vi "test_libssh2_userauth_keyboard_interactive_ex.vi"() -> ()   [LabVIEW 2013, in "libssh2_integration_tests.lvlib"]
uses:
  libssh2_integration_tests.lvlib
  callback_lvssh2_userauth_keyboard_interactive_response_function.vi
  libssh2/libssh2_init_default.vi
  libssh2/libssh2_session_handshake_tcp.vi
  libssh2/libssh2.lvlib
  <vilib>/addons/_JKI Toolkits/Caraya/classes/Test/Test.lvclass
  <vilib>/addons/_JKI Toolkits/Caraya/classes/Assert/Assert.lvclass
panel:
  out "error out":errorcluster
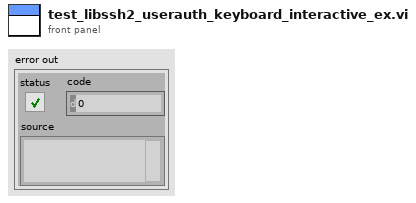
[diagram p1: front panel]
types:
  T1 = typedef "libssh2.lvlib/Session Refnum.ctl" = refnum<k1>
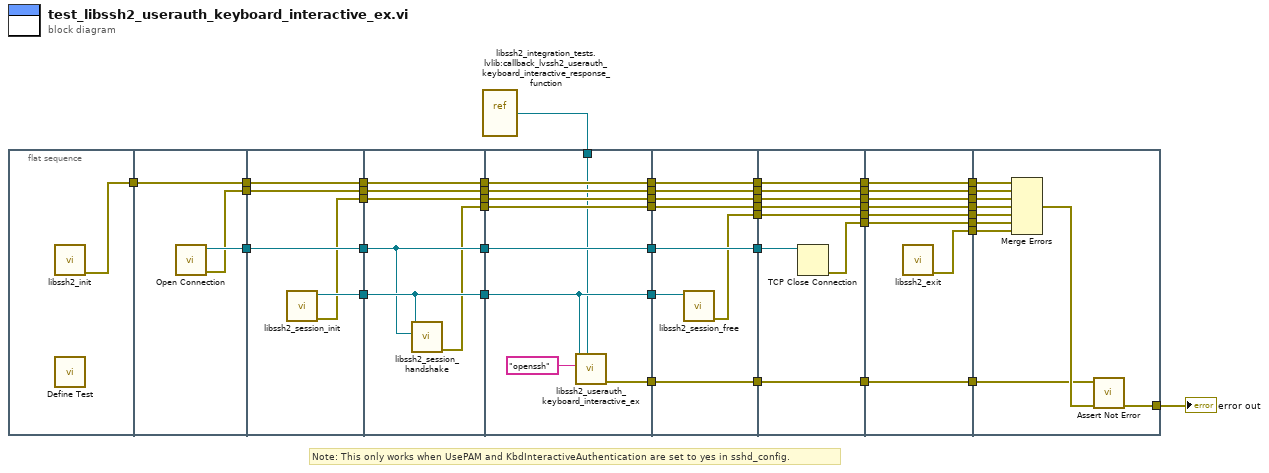
[diagram p0: block diagram]
diagram:
  # "Note: This only works when UsePAM and KbdInteractiveAuthentication are set to yes in sshd_config."
  n1 = flat-sequence {
    tunnel: [w47] -> w46
    tunnel: [w50] -> w45
    tunnel: w46 -> [w49]
    tunnel: [w49] -> w44
    tunnel: [w48] -> w43
    tunnel: w45 -> [w55]
    tunnel: [w55] -> w16
    tunnel: w44 -> [w54]
    tunnel: [w54] -> w15
    tunnel: w43 -> [w53]
    tunnel: [w53] -> w14
    tunnel: [w52] -> w13
    tunnel: [w51] -> w12
    tunnel: w16 -> [w57]
    tunnel: [w57] -> w31
    tunnel: w15 -> [w61]
    tunnel: [w61] -> w30
    tunnel: w14 -> [w60]
    tunnel: [w60] -> w29
    tunnel: [w59] -> w28
    tunnel: w13 -> [w59]
    tunnel: w12 -> [w58]
    tunnel: [w58] -> w27
    tunnel: [w56] -> w26
    tunnel: w31 -> [w70]
    tunnel: [w70] -> w8
    tunnel: w30 -> [w69]
    tunnel: [w69] -> w7
    tunnel: w29 -> [w68]
    tunnel: [w68] -> w6
    tunnel: w28 -> [w65]
    tunnel: w27 -> [w67]
    tunnel: [w67] -> w5
    tunnel: w26 -> [w66]
    tunnel: [w66] -> w4
    tunnel: [w65] -> w3
    tunnel: [w63] -> w2
    tunnel: w1 -> [w62]
    tunnel: w8 -> [w78]
    tunnel: [w78] -> w25
    tunnel: w7 -> [w77]
    tunnel: [w77] -> w24
    tunnel: w6 -> [w76]
    tunnel: [w76] -> w23
    tunnel: w5 -> [w75]
    tunnel: [w75] -> w22
    tunnel: w4 -> [w74]
    tunnel: [w74] -> w21
    tunnel: [w73] -> w18
    tunnel: [w72] -> w9
    tunnel: w2 -> [w72]
    tunnel: w3 -> [w71]
    tunnel: w25 -> [w86]
    tunnel: w24 -> [w85]
    tunnel: [w85] -> w42
    tunnel: w23 -> [w84]
    tunnel: [w84] -> w41
    tunnel: [w83] -> w40
    tunnel: w22 -> [w82]
    tunnel: [w82] -> w39
    tunnel: w21 -> [w81]
    tunnel: [w81] -> w38
    tunnel: [w80] -> w19
    tunnel: w18 -> [w80]
    tunnel: [w79] -> w10
    tunnel: w9 -> [w79]
    tunnel: w42 -> [w94]
    tunnel: [w94] -> w37
    tunnel: w41 -> [w93]
    tunnel: [w93] -> w36
    tunnel: w40 -> [w92]
    tunnel: [w92] -> w35
    tunnel: [w91] -> w34
    tunnel: w39 -> [w90]
    tunnel: [w90] -> w33
    tunnel: w38 -> [w89]
    tunnel: [w89] -> w32
    tunnel: [w88] -> w20
    tunnel: w19 -> [w88]
    tunnel: [w87] -> w11
    tunnel: w10 -> [w87]
    tunnel: w37 -> [w104]
    tunnel: w36 -> [w103]
    tunnel: w35 -> [w102]
    tunnel: w34 -> [w101]
    tunnel: w33 -> [w100]
    tunnel: [w98] -> w17
    tunnel: w32 -> [w97]
    tunnel: w20 -> [w96]
    tunnel: w11 -> [w95]
    frame #0 {
      n2 = call-poly "libssh2_init.vi"() -> ("error out"=w47:errorcluster)  [unwired: 11 in]
      n3 = call <vilib>:"Define Test.vi"() -> ()  [unwired: 10 in, 2 out]
    }
    frame #1 {
      n4 = call "Open Connection.vi"() -> ("error out"=w48:errorcluster, "connection ID"=w50:refnum<k5>)  [unwired: 10 in]
    }
    frame #2 {
      n5 = call "libssh2_session_init.vi"() -> ("error out"=w51:errorcluster, "session"=w52:T1)  [unwired: 10 in]
    }
    frame #3 {
      n6 = call-poly "libssh2_session_handshake.vi"("tcp connection"=w57, "session"=w59) -> ("error out"=w56:errorcluster)  [unwired: 9 in]
    }
    frame #4 {
      n7 = call "libssh2_userauth_keyboard_interactive_ex.vi"("response"=w62, "username"="openssh", "session"=w65) -> ("error out"=w63:errorcluster)  [unwired: 8 in]
    }
    frame #5 {
      n8 = call "libssh2_session_free.vi"("session"=w71) -> ("error out"=w73:errorcluster)  [unwired: 10 in]
    }
    frame #6 {
      n9 = TCP Close Connection(connection ID=w86) -> (error out=w83:errorcluster)  [unwired: 2 in, 1 out]
    }
    frame #7 {
      n10 = call "libssh2_exit.vi"() -> ("error out"=w91:errorcluster)  [unwired: 11 in]
    }
    frame #8 {
      n11 = Merge Errors(w104, w103, w100, w97, w96, w102, w101) -> (w99:errorcluster)
      n12 = call <vilib>:"Assert Not Error.vi"("error in (no error)"=w99, "Not Error?"=w95) -> ("error out"=w98:errorcluster)  [unwired: 8 in, 1 out]
    }
  }
  n13 = vi-ref "libssh2_integration_tests.lvlib:callback_lvssh2_userauth_keyboard_interactive_response_function.vi"() -> (w1:refnum<vi>)
  "error out" <- w17
